vi "NavbalLabVIEW(15-5-21).vi"() -> ()   [LabVIEW 2010] (continued)
  out "Marker Phase":sgl[][](array[numeric])
  in  "Marker Listbox":i32(listbox)
  out "Ref Pt Plot":sgl[][](array[numeric])
  in  "# Runs":dbl=15.0
  out "Predicted Phase":dbl[](array[numeric])
  out "Predicted Mag":dbl[](array[numeric])
  out "Port Output Data":string[][](array[string])
  out "Stbd Output Data":string[][](array[string])
  out "Excel Output Array":string[][](array[string])
  in  "Menu Button 6":bool
  in  "Menu Button 4":bool
  in  "Menu Button 5":bool
  in  "Menu Button 3":bool
  in  "Menu Button 2":bool
  in  "Menu Button 1":bool
  out "time string":string="6:13:31 AM"
  out "date string":string="3/22/2014"
  # "PORT"
  # "STARBOARD"
  # "120 Hz"
  # "60 Hz"
  # "Aft Turb"
  # "Aft Turb"
  # "Fwd Turb"
  # "Fwd Turb"
  # "Aft Gen"
  # "Aft Gen"
  # "Fwd Gen"
  # "Fwd Gen"
  # "NOTE: Use IMI Calibrator and\nmake sure dip switch in 'Peak' position"
  # "Simulated Signals Settings"
  # "NOTE: Each row is a different channel, columns correspond to rotational frequencies"
  # "NOTE: Each row is a different channel, columns correspond to rotational frequencies"
  # "NOTE: Each row is a different channel, columns correspond to rotational frequencies"
  # "NOTE: Each row is a different channel, columns correspond to rotational frequencies"
  # "FWD\nTURBINE"
  # "AFT \nGENERATOR"
  # "FWD\nGENERATOR"
  # "AFT\nTURBINE"
  # "START POINT"
  # "Weight"
  # "Location"
  # "Weight"
  # "Location"
  # "Weight"
  # "Location"
  # "Weight"
  # "Location"
  # "Weight"
  # "Location"
  # "Mag"
  # "Phase"
  # "Mag"
  # "Phase"
  # "Mag"
  # "Phase"
  # "Mag"
  # "Phase"
  # "Mag"
  # "Phase"
  # "Include how many runs in listbox?"
  # "3. Click \"Calculate Solution\"\n4. Double click desired solution option"
  # "1. Click  \"Calculate Response Coefficients\""
  # "2. Select Start Point"
  # "AT"
  # "AT"
  # "FT"
  # "FT"
  # "AG"
  # "AG"
  # "FG"
  # "FG"
  # "NET"
  # "Press to\nCalc Sum"
  # "AT"
  # "AT"
  # "AT"
  # "+"
  # "FT"
  # "FT"
  # "FT"
  # "LA: 10\nOhio: 2\nRig: 2 or 1"
  # "AG"
  # "AG"
  # "AG"
  # "FG"
  # "FG"
  # "FG"
  # "Sensor Weighting"
  # "AT              FT             AG             FG"
  # "AT             FT              AG             FG"
  # "Weight 1"
  # "Loc 2"
  # "Loc 1"
  # "Weight 2"
  # "Aft Turb"
  # "Fwd Turb"
  # "Aft Gen"
  # "Fwd Gen"
  # "Current"
  # "Marker"
  # "Solution"
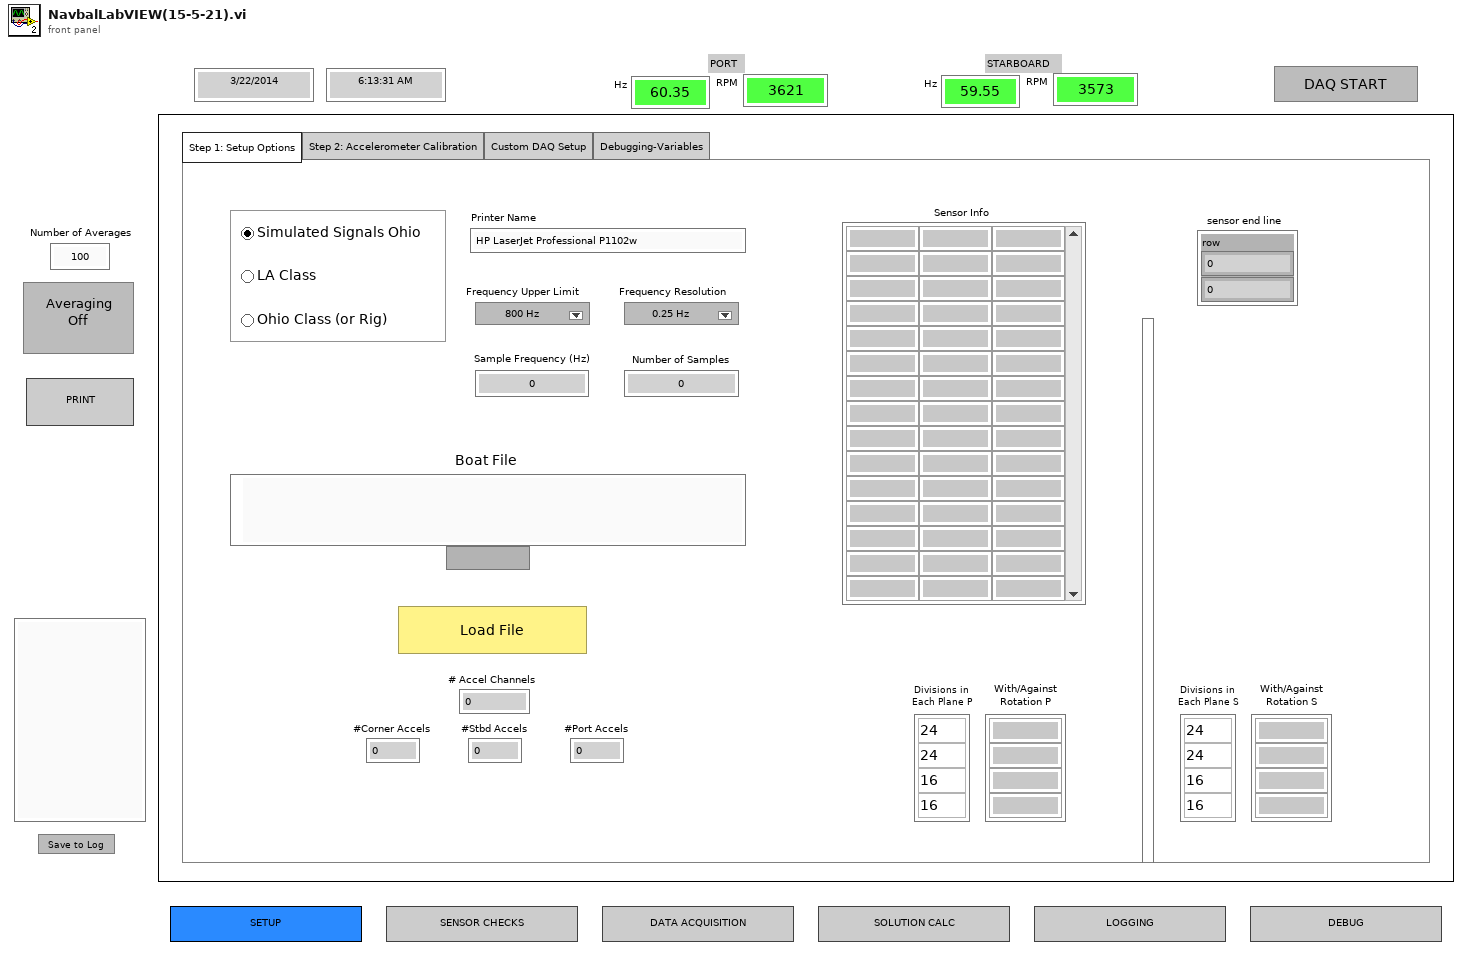
[diagram p1: front panel]
types:
  T1 = enum32{"Step 3: Background Checks", "Step 4: Sensor Overview", "Step 5: Vibration Survey", "Debugging - Indicators"}
  T2 = enum32{"Step 1: Setup Options", "Step 2: Accelerometer Calibration", "Custom DAQ Setup", "Debugging-Variables"}
  T3 = typedef "NI_Matrix.lvlib/RealMatrix.ctl" = dbl[][]
  T4 = enum32{"Simulated Signals Ohio", "LA Class", "Ohio Class"}
  T5 = cluster{"Amplitude":dbl, "Phase":dbl, "Amplitude 2":dbl, "Phase 2":dbl, "Amplitude 3":dbl, "Phase 3":dbl, "Amplitude 4":dbl, "Phase 4":dbl, "Amplitude 5":dbl, "Phase 5":dbl, "Amplitude 6":dbl, "Phase 6":dbl, "Amplitude 7":dbl, "Phase 7":dbl, "Amplitude 8":dbl, "Phase 8":dbl, "Amplitude 9":dbl, "Phase 9":dbl, "Amplitude 10":dbl, "Phase 10":dbl, "Amplitude 11":dbl, "Phase 11":dbl, "Amplitude 12":dbl, "Phase 12":dbl}
  T6 = cluster{"Frequency":dbl, "Amplitude":dbl, "Amplitude 2":dbl, "Amplitude 3":dbl, "Amplitude 4":dbl, "Amplitude 5":dbl, "Amplitude 6":dbl, "Amplitude 7":dbl, "Amplitude 8":dbl, "Amplitude 9":dbl, "Phase":dbl, "Phase 2":dbl, "Phase 3":dbl, "Phase 4":dbl, "Phase 5":dbl, "Phase 6":dbl, "Phase 7":dbl, "Phase 8":dbl, "Phase 9":dbl}
  T7 = enum32{"Other Adjustments", "Data Array STBD", "Data Array Port", "Data Array Corners-Stbd", "Data Array Corners-Port", "Solution Indicators", "Other Variables"}
  T8 = enum32{"Step 1: Response Coeff Variables", "Step 2: Calculate Goodman Solution", "Step 3: Optimal Balance Move", "Options", "Variables-For Reference"}
  T9 = enum32{"Step 6: Polar Plots", "Options", "Data Arrays"}
  T10 = cluster{"maximum":dbl, "minimum":dbl, "clip to min":bool, "log?(F)":bool, "grid color":u32, "plot color":u32, "fmt and prec":cluster{"format":enum8{"Decimal", "Scientific", "Engineering", "Binary", "Octal", "Hex"}, "precision":u8}, "visible section":u16}
  T11 = enum16{"Standard Report", "HTML", "Word", "Excel"}
  T12 = typedef "NI_ReportGenerationCore.lvlib/HTML Report Image Alignment.ctl" = enum16{"(default)", "LEFT", "RIGHT", "TOP", "TEXTTOP", "MIDDLE", "ABSMIDDLE", "BASELINE", "BOTTOM", "ABSBOTTOM"}
  T13 = cluster{"top":dbl, "left":dbl, "right":dbl, "bottom":dbl}
  T14 = cluster{"position (Excel)":cluster{"row":i32, "column":i32}, "name (Excel)":string, "bookmark (Word)":string}
  T15 = typedef "NI_Matrix.lvlib/ComplexMatrix.ctl" = cdb[][]
  T16 = enum8{"Enabled", "Disabled", "Disabled and Grayed Out"}
  T17 = typedef "Circular Buffer.lvlib/Circular Buffer Operations.ctl" = enum16{"Initialize", "Get Backlog", "Write", "Read (continuous)", "Read (most recent)"}
  T18 = typedef "NI_ReportGenerationToolkit.lvlib/font.ctl" = cluster{"font name":string, "font size":dbl, "bold":u16, "italic":u16, "underline":u16, "strike through":u16, "font color":u32}
  T19 = enum32{"Step 6: Polar Plots", "Data Arrays", "Options"}
  T20 = enum32{"Step 3: Sensor Overview", "Step 4: Background Checks", "Step 5: Vibration Survey", "Debugging - Indicators"}
  T21 = enum16{"User-specified Font", "Application Font", "System Font", "Dialog Font"}
  T22 = cluster{"Real Matrix Element":dbl, "Real Matrix Element":dbl}
  T23 = cluster{"Real Matrix Element":dbl, "Real Matrix Element":dbl}[]
  T24 = cluster{"Samples per Channel":u32, "# Accel Channels":i32}
diagram:
  w9 = u32 16252832
  # "random UI elements"
  # "Selection Color for Listbox"
  # "Default Booleans on Start"
  # "TODO:\nAdd Corner Pickups to both Starboard and Port Accel Arrays\n\nEdit Solution Permutation Structures for <4 plane Solutions\n\nAllow Solution Indicators to automatically grow to required dimensions as values are passed to them (Weights, Response Coeff, Prediction, etc.)\n\nMoving average indicator for last Scans, so that we can see more of the past scans\n->Add a Control for number of runs to average per point\n\nFull Implementation / Memory of recent Starboard and Port Baselines and Effects\n\nAllow Frequency indicator to update faster\n\n10/24/14\n- transferred from this computer to the Dell 1 computer (primary navbal computer)\n-"
  n1 = while {
    stop <- "stop 4" stop-if-true
    # "Event Structure: Button Nodes, Printer"
    n2 = control-ref of="Tab 1"() -> (w26:refnum<vi>)
    n3 = control-ref of="Tab 2"() -> (w13:refnum<vi>)
    n4 = control-ref of="Tab 3"() -> (w25:refnum<vi>)
    n5 = control-ref of="Tab 4"() -> (w24:refnum<vi>)
    n6 = control-ref of="Tab 5"() -> (w23:refnum<vi>)
    n7 = control-ref of="Tab 6"() -> (w22:refnum<vi>)
    n8 = Wait (ms)(milliseconds to wait=u32 500) -> ()  [unwired: 1 out]
    n9 = control-ref of="Menu Button 1"() -> (w21:refnum<vi>)
    n10 = control-ref of="Menu Button 2"() -> (w20:refnum<vi>)
    n11 = control-ref of="Menu Button 3"() -> (w19:refnum<vi>)
    n12 = control-ref of="Menu Button 5"() -> (w18:refnum<vi>)
    n13 = control-ref of="Menu Button 4"() -> (w17:refnum<vi>)
    n14 = control-ref of="Menu Button 6"() -> (w16:refnum<vi>)
    n15 = event shown="[4] \"Solution Options\": Value Change" {
      selector: _ -> [_ _ _ _ _ _ _ _ _ _ _ _ _ _ _ _ _ _]
      dyn-events: _ -> [_ _ _ _ _ _ _ _ _ _ _ _ _ _ _ _ _ _]
      timeout: _ -> [_ _ _ _ _ _ _ _ _ _ _ _ _ _ _ _ _ _]
      tunnel: w26 -> [w37 w57 w77 w97 _ _ _ _ _ _ _ w206 w225 w252 _ _ _ _]
      tunnel: w25 -> [w46 w66 w86 w106 _ _ _ _ _ _ _ w215 w235 w250 _ _ _ _]
      tunnel: w24 -> [w45 w65 w85 w105 _ _ _ _ _ _ _ w214 w234 w249 _ _ _ _]
      tunnel: w23 -> [w44 w64 w84 w104 _ _ _ _ _ _ _ w213 w233 w248 _ _ _ _]
      tunnel: w22 -> [w43 w63 w83 w103 _ _ _ _ _ _ _ w212 w232 w247 _ _ _ _]
      tunnel: w21 -> [w34 w56 w76 w96 _ _ _ _ _ _ _ w205 w224 _ _ _ _ _]
      tunnel: w20 -> [w33 w55 w75 w95 _ _ _ _ _ _ _ w204 w223 _ _ _ _ _]
      tunnel: w19 -> [w32 w54 w74 w94 _ _ _ _ _ _ _ w203 w222 _ _ _ _ _]
      tunnel: w18 -> [w31 w53 w73 w93 _ _ _ _ _ _ _ w202 w221 _ _ _ _ _]
      tunnel: w17 -> [w30 w52 w72 w92 _ _ _ _ _ _ _ w201 w220 _ _ _ _ _]
      tunnel: w16 -> [w29 w51 w71 w91 _ _ _ _ _ _ _ w200 w219 _ _ _ _ _]
      tunnel: "Printer Name" -> [_ _ _ _ _ _ _ _ _ _ _ _ _ w266 _ _ _ _]
      tunnel: w13 -> [w27 w47 w67 w87 _ _ _ _ _ _ _ w196 w216 w251 _ _ _ _]
      event "Menu Button 1": Value Change {
        w35 = cluster{u32, u32}[] [{6579300, 13421772}] ("Colors [4]")
        n16 = event-data() -> ()  [unwired: 1 in, 5 out]
        n17 = property on="Property Node" class="TabCtl (strict)"(reference=w43, "Visible"=FALSE) -> ()  [unwired: 1 in, 2 out]
        n18 = property on="Property Node" class="TabCtl (strict)"(reference=w44, "Visible"=FALSE) -> ()  [unwired: 1 in, 2 out]
        n19 = property on="Property Node" class="TabCtl (strict)"(reference=w37, "Visible"=TRUE) -> ()  [unwired: 1 in, 2 out]
        n20 = property on="Property Node" class="TabCtl (strict)"(reference=w45, "Visible"=FALSE) -> ()  [unwired: 1 in, 2 out]
        n21 = property on="Property Node" class="TabCtl (strict)"(reference=w27, "Visible"=FALSE) -> ()  [unwired: 1 in, 2 out]
        n22 = property on="Property Node" class="TabCtl (strict)"(reference=w46, "Visible"=FALSE) -> ()  [unwired: 1 in, 2 out]
        n23 = property on="Property Node" class="Bool"(reference=w34, "Colors [4]"=cluster{u32, u32}[] [{0, 2788095}, {0, 0}, {0, 11513775}, {0, 0}]) -> ()  [unwired: 1 in, 2 out]
        n24 = property on="Property Node" class="Bool"(reference=w31, "Colors [4]"=w35) -> ()  [unwired: 1 in, 2 out]
        n25 = property on="Property Node" class="Bool"(reference=w30, "Colors [4]"=w35) -> ()  [unwired: 1 in, 2 out]
        n26 = property on="Property Node" class="Bool"(reference=w29, "Colors [4]"=w35) -> ()  [unwired: 1 in, 2 out]
        n27 = property on="Property Node" class="Bool"(reference=w33, "Colors [4]"=w35) -> ()  [unwired: 1 in, 2 out]
        n28 = property on="Property Node" class="Bool"(reference=w32, "Colors [4]"=w35) -> ()  [unwired: 1 in, 2 out]
      }
      event "Menu Button 2": Value Change {
        w49 = cluster{u32, u32}[] [{6579300, 13421772}] ("Colors [4]")
        n29 = event-data() -> ()  [unwired: 1 in, 5 out]
        n30 = property on="Property Node" class="TabCtl (strict)"(reference=w63, "Visible"=FALSE) -> ()  [unwired: 1 in, 2 out]
        n31 = property on="Property Node" class="TabCtl (strict)"(reference=w64, "Visible"=FALSE) -> ()  [unwired: 1 in, 2 out]
        n32 = property on="Property Node" class="TabCtl (strict)"(reference=w57, "Visible"=FALSE) -> ()  [unwired: 1 in, 2 out]
        n33 = property on="Property Node" class="TabCtl (strict)"(reference=w47, "Visible"=TRUE) -> ()  [unwired: 1 in, 2 out]
        n34 = property on="Property Node" class="TabCtl (strict)"(reference=w65, "Visible"=FALSE) -> ()  [unwired: 1 in, 2 out]
        n35 = property on="Property Node" class="TabCtl (strict)"(reference=w66, "Visible"=FALSE) -> ()  [unwired: 1 in, 2 out]
        n36 = property on="Property Node" class="Bool"(reference=w56, "Colors [4]"=w49) -> ()  [unwired: 1 in, 2 out]
        n37 = property on="Property Node" class="Bool"(reference=w53, "Colors [4]"=w49) -> ()  [unwired: 1 in, 2 out]
        n38 = property on="Property Node" class="Bool"(reference=w52, "Colors [4]"=w49) -> ()  [unwired: 1 in, 2 out]
        n39 = property on="Property Node" class="Bool"(reference=w55, "Colors [4]"=cluster{u32, u32}[] [{0, 16753194}, {0, 0}, {0, 11513775}, {0, 0}]) -> ()  [unwired: 1 in, 2 out]
        n40 = property on="Property Node" class="Bool"(reference=w51, "Colors [4]"=w49) -> ()  [unwired: 1 in, 2 out]
        n41 = property on="Property Node" class="Bool"(reference=w54, "Colors [4]"=w49) -> ()  [unwired: 1 in, 2 out]
      }
      event "Menu Button 3": Value Change {
        w69 = cluster{u32, u32}[] [{6579300, 13421772}] ("Colors [4]")
        n42 = event-data() -> ()  [unwired: 1 in, 5 out]
        n43 = property on="Property Node" class="TabCtl (strict)"(reference=w83, "Visible"=FALSE) -> ()  [unwired: 1 in, 2 out]
        n44 = property on="Property Node" class="TabCtl (strict)"(reference=w84, "Visible"=FALSE) -> ()  [unwired: 1 in, 2 out]
        n45 = property on="Property Node" class="TabCtl (strict)"(reference=w77, "Visible"=FALSE) -> ()  [unwired: 1 in, 2 out]
        n46 = property on="Property Node" class="TabCtl (strict)"(reference=w85, "Visible"=FALSE) -> ()  [unwired: 1 in, 2 out]
        n47 = property on="Property Node" class="TabCtl (strict)"(reference=w67, "Visible"=FALSE) -> ()  [unwired: 1 in, 2 out]
        n48 = property on="Property Node" class="TabCtl (strict)"(reference=w86, "Visible"=TRUE) -> ()  [unwired: 1 in, 2 out]
        n49 = property on="Property Node" class="Bool"(reference=w76, "Colors [4]"=w69) -> ()  [unwired: 1 in, 2 out]
        n50 = property on="Property Node" class="Bool"(reference=w73, "Colors [4]"=w69) -> ()  [unwired: 1 in, 2 out]
        n51 = property on="Property Node" class="Bool"(reference=w72, "Colors [4]"=w69) -> ()  [unwired: 1 in, 2 out]
        n52 = property on="Property Node" class="Bool"(reference=w75, "Colors [4]"=w69) -> ()  [unwired: 1 in, 2 out]
        n53 = property on="Property Node" class="Bool"(reference=w71, "Colors [4]"=w69) -> ()  [unwired: 1 in, 2 out]
        n54 = property on="Property Node" class="Bool"(reference=w74, "Colors [4]"=cluster{u32, u32}[] [{0, 16025855}, {0, 0}, {0, 11513775}, {0, 0}]) -> ()  [unwired: 1 in, 2 out]
      }
      event "Menu Button 4": Value Change {
        w90 = cluster{u32, u32}[] [{6579300, 13421772}] ("Colors [4]")
        n55 = event-data() -> ()  [unwired: 1 in, 5 out]
        n56 = property on="Property Node" class="TabCtl (strict)"(reference=w103, "Visible"=FALSE) -> ()  [unwired: 1 in, 2 out]
        n57 = property on="Property Node" class="TabCtl (strict)"(reference=w104, "Visible"=TRUE) -> ()  [unwired: 1 in, 2 out]
        n58 = property on="Property Node" class="TabCtl (strict)"(reference=w97, "Visible"=FALSE) -> ()  [unwired: 1 in, 2 out]
        n59 = property on="Property Node" class="TabCtl (strict)"(reference=w87, "Visible"=FALSE) -> ()  [unwired: 1 in, 2 out]
        n60 = property on="Property Node" class="TabCtl (strict)"(reference=w105, "Visible"=FALSE) -> ()  [unwired: 1 in, 2 out]
        n61 = property on="Property Node" class="TabCtl (strict)"(reference=w106, "Visible"=FALSE) -> ()  [unwired: 1 in, 2 out]
        n62 = property on="Property Node" class="Bool"(reference=w96, "Colors [4]"=w90) -> ()  [unwired: 1 in, 2 out]
        n63 = property on="Property Node" class="Bool"(reference=w93, "Colors [4]"=w90) -> ()  [unwired: 1 in, 2 out]
        n64 = property on="Property Node" class="Bool"(reference=w92, "Colors [4]"=cluster{u32, u32}[] [{0, 2853120}, {0, 0}, {0, 11513775}, {0, 0}]) -> ()  [unwired: 1 in, 2 out]
        n65 = property on="Property Node" class="Bool"(reference=w95, "Colors [4]"=w90) -> ()  [unwired: 1 in, 2 out]
        n66 = property on="Property Node" class="Bool"(reference=w91, "Colors [4]"=w90) -> ()  [unwired: 1 in, 2 out]
        n67 = property on="Property Node" class="Bool"(reference=w94, "Colors [4]"=w90) -> ()  [unwired: 1 in, 2 out]
      }
      event "Solution Options": Value Change {
        w107 = string[][] []
        w108 = csg[] [] ("AT Exceptions")
        n68 = event-data() -> ()  [unwired: 1 in, 5 out]
        n69 = property on="Aft Turbine Balance Plane Split Options" class="MCListbox (strict)"("ItemNames"=w107) -> ()  [unwired: 2 in, 2 out]
        n70 = property on="Fwd Turbine Balance Plane Split Options" class="MCListbox (strict)"("ItemNames"=w107) -> ()  [unwired: 2 in, 2 out]
        n71 = for {
          N: 50 -> [_]
          i -> [w112]
          n72 = Bundle(w112, "Column"=3) -> (w111:cluster{i32, "Column":i32})  [unwired: 1 in]
          n73 = property on="Prediction Results" class="MCListbox (strict)"("ActiveCell"=w111) -> ()  [unwired: 2 in, 2 out]
          n74 = property on="Prediction Results" class="MCListbox (strict)"("CellBG"=u32 16777215) -> ()  [unwired: 2 in, 2 out]
        }
        n75 = property on="Solution Options" class="MCListbox (strict)"("SelColor"=u32 2771455) -> ()  [unwired: 2 in, 2 out]
        n76 = property on="Fwd Generator Balance Plane Split Options" class="MCListbox (strict)"("ItemNames"=w107) -> ()  [unwired: 2 in, 2 out]
        n77 = property on="Aft Generator Balance Plane Split Options" class="MCListbox (strict)"("ItemNames"=w107) -> ()  [unwired: 2 in, 2 out]
        n78 = local write "AT Exceptions"(w108) -> ()
        n79 = local write "FT Exceptions"(w108) -> ()
        n80 = local write "AG Exceptions"(w108) -> ()
        n81 = local write "FG Exceptions"(w108) -> ()
      }
      event "Weight Category AT": Value Change {
        n82 = event-data() -> ()  [unwired: 1 in, 5 out]
      }
      event "MagPhase": Mouse Down {
        n83 = event-data() -> ()  [unwired: 1 in, 7 out]
        n84 = for {
          N: 60 -> [_]
          i -> [w116]
          n85 = flat-sequence {
            tunnel: w116 -> [w119]
            frame #0 {
              n86 = Bundle(w119, 5) -> (w117:cluster{i32, i32})  [unwired: 1 in]
              n87 = property on="MagPhase" class="MCListbox (strict)"("ActiveCell"=w117) -> ()  [unwired: 2 in, 2 out]
            }
            frame #1 {
              n88 = property on="MagPhase" class="MCListbox (strict)"("CellBG"=u32 16777215) -> ()  [unwired: 2 in, 2 out]
            }
          }
        }
      }
      event "Weight Category FT": Value Change {
        n89 = event-data() -> ()  [unwired: 1 in, 5 out]
      }
      event "Weight Category AG": Value Change {
        n90 = event-data() -> ()  [unwired: 1 in, 5 out]
      }
      event "Weight Category FG": Value Change {
        n91 = event-data() -> ()  [unwired: 1 in, 5 out]
      }
      event "Load File": Value Change {
        w144 = 0
        # "Whether Planes are with or Against \nRotation"
        # "Number of Balance Plane Divisions:\n3rd tab 2nd row"
        # "Sensor info: Pick up the first \n3 columns from the  4th tab in Excel"
        n92 = event-data() -> ()  [unwired: 1 in, 5 out]
        n93 = property on="Boat File" class="Path"() -> ("Value"=w164:path)  [unwired: 2 in, 2 out]
        n94 = call <vilib>:"New Report.vi"("report type"=T11."Excel", "template (empty)"=w164) -> ("report out"=w157:refnum<class "NI_report.lvclass">, "error out"=w156:errorcluster)  [unwired: 12 in]
        n95 = call <vilib>:"Excel Get Worksheet.vi"("report in"=w157, "worksheet index (0)"=2, "error in (no error)"=w156) -> ("report out"=w136:refnum<class "NI_report.lvclass">, "error out"=w135:errorcluster)  [unwired: 11 out]
        n96 = call <vilib>:"Excel Get Worksheet.vi"("report in"=w157, "worksheet index (0)"=3, "error in (no error)"=w156) -> ("report out"=w152:refnum<class "NI_report.lvclass">, "error out"=w151:errorcluster)  [unwired: 11 out]
        n97 = call <vilib>:"Excel Get Last Row.vi"("report in"=w152, "error in (no error)"=w151) -> ("report out"=w160:refnum<class "NI_report.lvclass">, "MS Office parameters out"=w170:T14, "error out"=w159:errorcluster)  [unwired: 11 in]
        n98 = call-poly <vilib>:"Excel Get Data.vi"("report in"=w136, "data type"=string[][] [], "start (-1, -1)"=cluster{"row":i32, "column":i32} {"row"=2, "column"=1}, "end (-1, -1)"=cluster{"row":i32, "column":i32} {"row"=2, "column"=8} ("start (-1, -1)"), "error in (no error)"=w135) -> ("data"=w131:string[][])  [unwired: 10 out]
        n99 = call-poly <vilib>:"Excel Get Data.vi"("report in"=w136, "data type"=i32[][] [], "start (-1, -1)"=cluster{"row":i32, "column":i32} {"row"=1, "column"=1}, "end (-1, -1)"=cluster{"row":i32, "column":i32} {"row"=1, "column"=8} ("start (-1, -1)"), "error in (no error)"=w135) -> ("data"=w145:i32[][])  [unwired: 10 out]
        n100 = Unbundle(w170) -> ("position (Excel)"=w169:cluster{"row":i32, "column":i32})  [unwired: 2 out]
        n101 = Transpose 2D Array(2D array=w131) -> (transposed array=w126:string[][])
        n102 = Transpose Matrix(1:w145) -> (0:w130:dbl[][])
        n103 = Unbundle(w169) -> ("row"=w168:i32)  [unwired: 1 out]
        n104 = Decrement(x=w168) -> (x-1=w150:i32)
        n105 = Delete From Array(array=w130, length=4, index (row)=4 ("disabled index (col)")) -> (deleted portion=w128:dbl[][], array with subset deleted=w121:dbl[][])  [unwired: 1 in]
        n106 = Delete From Array(array=w126, length=4, index (row)=4 ("disabled index (col)")) -> (deleted portion=→"With/Against\nRotation S":string[][], array with subset deleted=→"With/Against\nRotation P":string[][])  [unwired: 1 in]
        n107 = Bundle(w150, 2) -> (w162:cluster{i32, i32})  [unwired: 1 in]
        "sensor end line" <- w162
        n108 = call-poly <vilib>:"Excel Get Data.vi"("report in"=w160, "data type"=string[][] [], "start (-1, -1)"=cluster{"row":i32, "column":i32} {"row"=1, "column"=0}, "end (-1, -1)"=w162, "error in (no error)"=w159) -> ("data"=w143:string[][], "error out"=w161:errorcluster)  [unwired: 9 out]
        "Sensor Info" <- w143
        n109 = call <vilib>:"General Error Handler.vi"("error in (no error)"=w161) -> ()  [unwired: 2 in, 13 out]
        n110 = Array Size(array=w143) -> (size(s)=w148:i32[])
        n111 = Array Size(array=w143) -> (size(s)=w142:i32[])
        n112 = Index Array(array=w148, index=0) -> (element=→"# Accel Channels":i32)
        n113 = property on="Divisions in\nEach Plane S" class="Arr (strict)"("Value"=w128) -> ()  [unwired: 2 in, 2 out]
        n114 = property on="Divisions in\nEach Plane P" class="Arr (strict)"("Value"=w121) -> ()  [unwired: 2 in, 2 out]
        n115 = Index Array(array=w142, index=0) -> (element=w140:i32)
        n116 = for {
          N: w140 -> [_]
          tunnel: w143 -> [w186]
          shift-right: [w180] -> w139
          shift-left: w144 -> [w181]
          shift-right: [w176] -> w138
          shift-left: w144 -> [w177]
          shift-right: [w174] -> w137
          shift-left: w144 -> [w175]
          i -> [w184]
          n117 = Index Array(array=w186, index (row)=w184, index (col)=2 ("disabled index (col)")) -> (element=w171:string)
          n118 = Equal?(x=w171, y="Corner") -> (x = y?=w182:bool)
          n119 = Equal?(x=w171, y="Stbd Brng") -> (x = y?=w178:bool)
          n120 = Equal?(x=w171, y="Port Brng") -> (x = y?=w172:bool)
          n121 = case shown="True" w182 {
            tunnel: w181 -> [w193 w195]
            tunnel: [w193 w194] -> w180
            frame False {
            }
            frame True {
              n122 = Increment(x=w195) -> (x+1=w194:i32)
            }
          }
          n123 = case shown="True" w178 {
            tunnel: [w190 w192] -> w176
            tunnel: w177 -> [w190 w191]
            frame False {
            }
            frame True {
              n124 = Increment(x=w191) -> (x+1=w192:i32)
            }
          }
          n125 = case shown="True" w172 {
            tunnel: [w187 w189] -> w174
            tunnel: w175 -> [w187 w188]
            frame False {
            }
            frame True {
              n126 = Increment(x=w188) -> (x+1=w189:i32)
            }
          }
        }
        "#Corner Accels" <- w139
        "#Stbd Accels" <- w138
        "#Port Accels" <- w137
      }
      event "Menu Button 5": Value Change {
        w199 = cluster{u32, u32}[] [{6579300, 13421772}] ("Colors [4]")
        n127 = event-data() -> ()  [unwired: 1 in, 5 out]
        n128 = property on="Property Node" class="TabCtl (strict)"(reference=w212, "Visible"=FALSE) -> ()  [unwired: 1 in, 2 out]
        n129 = property on="Property Node" class="TabCtl (strict)"(reference=w213, "Visible"=FALSE) -> ()  [unwired: 1 in, 2 out]
        n130 = property on="Property Node" class="TabCtl (strict)"(reference=w206, "Visible"=FALSE) -> ()  [unwired: 1 in, 2 out]
        n131 = property on="Property Node" class="TabCtl (strict)"(reference=w214, "Visible"=TRUE) -> ()  [unwired: 1 in, 2 out]
        n132 = property on="Property Node" class="TabCtl (strict)"(reference=w196, "Visible"=FALSE) -> ()  [unwired: 1 in, 2 out]
        n133 = property on="Property Node" class="TabCtl (strict)"(reference=w215, "Visible"=FALSE) -> ()  [unwired: 1 in, 2 out]
        n134 = property on="Property Node" class="Bool"(reference=w205, "Colors [4]"=w199) -> ()  [unwired: 1 in, 2 out]
        n135 = property on="Property Node" class="Bool"(reference=w202, "Colors [4]"=cluster{u32, u32}[] [{0, 13696881}, {0, 0}, {0, 11513775}, {0, 0}]) -> ()  [unwired: 1 in, 2 out]
        n136 = property on="Property Node" class="Bool"(reference=w201, "Colors [4]"=w199) -> ()  [unwired: 1 in, 2 out]
        n137 = property on="Property Node" class="Bool"(reference=w204, "Colors [4]"=w199) -> ()  [unwired: 1 in, 2 out]
        n138 = property on="Property Node" class="Bool"(reference=w200, "Colors [4]"=w199) -> ()  [unwired: 1 in, 2 out]
        n139 = property on="Property Node" class="Bool"(reference=w203, "Colors [4]"=w199) -> ()  [unwired: 1 in, 2 out]
      }
      event "Menu Button 6": Value Change {
        w218 = cluster{u32, u32}[] [{6579300, 13421772}] ("Colors [4]")
        n140 = event-data() -> ()  [unwired: 1 in, 5 out]
        n141 = property on="Property Node" class="TabCtl (strict)"(reference=w232, "Visible"=TRUE) -> ()  [unwired: 1 in, 2 out]
        n142 = property on="Property Node" class="TabCtl (strict)"(reference=w233, "Visible"=FALSE) -> ()  [unwired: 1 in, 2 out]
        n143 = property on="Property Node" class="TabCtl (strict)"(reference=w225, "Visible"=FALSE) -> ()  [unwired: 1 in, 2 out]
        n144 = property on="Property Node" class="TabCtl (strict)"(reference=w216, "Visible"=FALSE) -> ()  [unwired: 1 in, 2 out]
        n145 = property on="Property Node" class="TabCtl (strict)"(reference=w234, "Visible"=FALSE) -> ()  [unwired: 1 in, 2 out]
        n146 = property on="Property Node" class="TabCtl (strict)"(reference=w235, "Visible"=FALSE) -> ()  [unwired: 1 in, 2 out]
        n147 = property on="Property Node" class="Bool"(reference=w224, "Colors [4]"=w218) -> ()  [unwired: 1 in, 2 out]
        n148 = property on="Property Node" class="Bool"(reference=w221, "Colors [4]"=w218) -> ()  [unwired: 1 in, 2 out]
        n149 = property on="Property Node" class="Bool"(reference=w220, "Colors [4]"=w218) -> ()  [unwired: 1 in, 2 out]
        n150 = property on="Property Node" class="Bool"(reference=w223, "Colors [4]"=w218) -> ()  [unwired: 1 in, 2 out]
        n151 = property on="Property Node" class="Bool"(reference=w219, "Colors [4]"=cluster{u32, u32}[] [{0, 5888767}, {0, 0}, {0, 11513775}, {0, 0}]) -> ()  [unwired: 1 in, 2 out]
        n152 = property on="Property Node" class="Bool"(reference=w222, "Colors [4]"=w218) -> ()  [unwired: 1 in, 2 out]
      }
      event "Print Button": Value Change {
        w267 = 1 items=["portrait", "landscape"] ("orientation (portrait)")
        n153 = event-data() -> ()  [unwired: 1 in, 5 out]
        n154 = property on="Tab 1" class="TabCtl (strict)"() -> ("Visible"=w246:bool)  [unwired: 2 in, 2 out]
        n155 = property on="Tab 2" class="TabCtl (strict)"() -> ("Visible"=w245:bool)  [unwired: 2 in, 2 out]
        n156 = property on="Tab 3" class="TabCtl (strict)"() -> ("Visible"=w241:bool)  [unwired: 2 in, 2 out]
        n157 = property on="Tab 4" class="TabCtl (strict)"() -> ("Visible"=w242:bool)  [unwired: 2 in, 2 out]
        n158 = property on="Tab 5" class="TabCtl (strict)"() -> ("Visible"=w243:bool)  [unwired: 2 in, 2 out]
        n159 = property on="Tab 6" class="TabCtl (strict)"() -> ("Visible"=w244:bool)  [unwired: 2 in, 2 out]
        n160 = Build Array(w252, w251, w250, w249, w248, w247) -> (w238:refnum<vi>[])
        n161 = Build Array(w246, w245, w241, w242, w243, w244) -> (w240:bool[])
        n162 = call <vilib>:"New Report.vi"("report type"=T11."Standard Report") -> ("report out"=w274:refnum<class "NI_report.lvclass">, "error out"=w273:errorcluster)  [unwired: 13 in]
        n163 = Get Date/Time String(want seconds? (F)=TRUE) -> (date string=w256:string, time string=w255:string)  [unwired: 2 in]
        n164 = for {
          tunnel: w240 -> [w277] mode=indexing
          tunnel: [w275] -> w239 mode=indexing
          i -> [w276]
          n165 = case shown="True" w277 {
            tunnel: w276 -> [_ w279]
            tunnel: [-1 w279] -> w275
            frame False {
            }
            frame True {
            }
          }
        }
        n166 = Concatenate Strings(w256, " - " ("string"), w255) -> (w253:string)
        n167 = Array Max & Min(array=w239) -> (max value=w237:i32)  [unwired: 3 out]
        n168 = Index Array(array=w238, index=w237) -> (element=w236:refnum<vi>)
        n169 = call-dynamic "Append Control Image to Report.vi"("report in"=w274, "alignment (default)"=HTML_Report_Image_Alignment."MIDDLE", "ctrl reference"=w236, "error in (no error)"=w273) -> ("report out"=w269:refnum<class "NI_report.lvclass">, "error out"=w268:errorcluster)  [unwired: 8 in, 2 out]
        n170 = call-dynamic "Set Report Orientation.vi"("report in"=w269, "orientation (portrait)"=w267, "error in (no error)"=w268) -> ("report out"=w264:refnum<class "NI_report.lvclass">, "error out"=w265:errorcluster)  [unwired: 11 in]
        n171 = call-dynamic "Set Report Margins.vi"("report in"=w264, "margins (1.00)"=T13 {"top"=0.3, "left"=0.5, "right"=0.5, "bottom"=0.3}, "error in (no error)"=w265) -> ("report out"=w262:refnum<class "NI_report.lvclass">, "error out"=w261:errorcluster)  [unwired: 10 in, 1 out]
        n172 = call-dynamic "Set Report Footer Text.vi"("report in"=w262, "center footer text"=w253, "error in (no error)"=w261) -> ("report out"=w260:refnum<class "NI_report.lvclass">, "error out"=w259:errorcluster)  [unwired: 11 in]
        n173 = call-dynamic "Print Report.vi"("report in"=w260, "printer name (default)"=w266, "error in (no error)"=w259) -> ("report out"=w272:refnum<class "NI_report.lvclass">, "error out"=w271:errorcluster)  [unwired: 11 in]
        n174 = call-dynamic "Dispose Report.vi"("report in"=w272, "error in (no error)"=w271) -> ()  [unwired: 13 in, 1 out]
      }
      event "Aft Turbine Balance Plane Split Options": Value Change {
        n175 = event-data() -> ()  [unwired: 1 in, 5 out]
        n176 = for {
          N: 50 -> [_]
          i -> [w283]
          n177 = Bundle(w283, "Column"=3) -> (w282:cluster{i32, "Column":i32})  [unwired: 1 in]
          n178 = property on="Prediction Results" class="MCListbox (strict)"("ActiveCell"=w282) -> ()  [unwired: 2 in, 2 out]
          n179 = property on="Prediction Results" class="MCListbox (strict)"("CellBG"=u32 16777215) -> ()  [unwired: 2 in, 2 out]
        }
        n180 = property on="Aft Turbine Balance Plane Split Options" class="MCListbox (strict)"("SelColor"=u32 2771455) -> ()  [unwired: 2 in, 2 out]
      }
      event "Fwd Turbine Balance Plane Split Options": Value Change {
        n181 = event-data() -> ()  [unwired: 1 in, 5 out]
        n182 = for {
          N: 50 -> [_]
          i -> [w289]
          n183 = Bundle(w289, "Column"=3) -> (w288:cluster{i32, "Column":i32})  [unwired: 1 in]
          n184 = property on="Prediction Results" class="MCListbox (strict)"("ActiveCell"=w288) -> ()  [unwired: 2 in, 2 out]
          n185 = property on="Prediction Results" class="MCListbox (strict)"("CellBG"=u32 16777215) -> ()  [unwired: 2 in, 2 out]
        }
        n186 = property on="Fwd Turbine Balance Plane Split Options" class="MCListbox (strict)"("SelColor"=u32 2771455) -> ()  [unwired: 2 in, 2 out]
      }
      event "Aft Generator Balance Plane Split Options": Value Change {
        n187 = event-data() -> ()  [unwired: 1 in, 5 out]
        n188 = for {
          N: 50 -> [_]
          i -> [w295]
          n189 = Bundle(w295, "Column"=3) -> (w294:cluster{i32, "Column":i32})  [unwired: 1 in]
          n190 = property on="Prediction Results" class="MCListbox (strict)"("ActiveCell"=w294) -> ()  [unwired: 2 in, 2 out]
          n191 = property on="Prediction Results" class="MCListbox (strict)"("CellBG"=u32 16777215) -> ()  [unwired: 2 in, 2 out]
        }
        n192 = property on="Aft Generator Balance Plane Split Options" class="MCListbox (strict)"("SelColor"=u32 2771455) -> ()  [unwired: 2 in, 2 out]
      }
      event "Fwd Generator Balance Plane Split Options": Value Change {
        n193 = event-data() -> ()  [unwired: 1 in, 5 out]
        n194 = for {
          N: 50 -> [_]
          i -> [w301]
          n195 = Bundle(w301, "Column"=3) -> (w300:cluster{i32, "Column":i32})  [unwired: 1 in]
          n196 = property on="Prediction Results" class="MCListbox (strict)"("ActiveCell"=w300) -> ()  [unwired: 2 in, 2 out]
          n197 = property on="Prediction Results" class="MCListbox (strict)"("CellBG"=u32 16777215) -> ()  [unwired: 2 in, 2 out]
        }
        n198 = property on="Fwd Generator Balance Plane Split Options" class="MCListbox (strict)"("SelColor"=u32 2771455) -> ()  [unwired: 2 in, 2 out]
      }
    }
  }
  n199 = while {
    stop <- "stop 2" stop-if-true
    w305 = path "C:/Users/Jim Gehringer/Desktop/Navbal-LabVIEW_FINAL/Balancelog.txt" ("file (use dialog)")
    # "Logging"
    # "Time and Date"
    n200 = call <vilib>:"Check if File or Folder Exists.vi"("path"=w305) -> ("file or folder exists?"=w315:bool)  [unwired: 8 in, 2 out]
    n201 = Get Date/Time String(want seconds? (F)=TRUE) -> (date string=w304:string, time string=w316:string)  [unwired: 2 in]
    "date string" <- w304
    "time string" <- w316
    n202 = case shown="True" w315 {
      tunnel: w305 -> [_ w340]
      frame False {
      }
      frame True {
        n203 = Read from Text File(file (use dialog)=w340) -> (text=→"text":string)  [unwired: 3 in, 3 out]
      }
    }
    n204 = case shown="True" "Enter into log" {
      tunnel: w316 -> [_ w324]
      tunnel: w305 -> [_ w321]
      tunnel: w304 -> [_ w319]
      frame False {
      }
      frame True {
        n205 = call <vilib>:"Check if File or Folder Exists.vi"("path"=w321) -> ("file or folder exists?"=w323:bool)  [unwired: 8 in, 2 out]
        n206 = property on="Log Input" class="Str"("Value"="" ("Log Input")) -> ()  [unwired: 2 in, 2 out]
        n207 = case shown="True" w323 {
          tunnel: w321 -> [w327 w337]
          tunnel: w324 -> [w331 w334]
          tunnel: "Log Input" -> [w329 w336]
          tunnel: w319 -> [w325 w332]
          frame False {
            n208 = call <vilib>:"Space Constant.vi"() -> ("String"=w326:string)
            n209 = Concatenate Strings(w325, w326, w331, "\r", w329) -> (w328:string)
            n210 = Write to Text File(file (use dialog)=w327, text=w328) -> ()  [unwired: 2 in, 3 out]
          }
          frame True {
            w335 = "\r"
            n211 = call <vilib>:"Space Constant.vi"() -> ("String"=w333:string)
            n212 = Read from Text File(file (use dialog)=w337) -> (text=w339:string)  [unwired: 3 in, 3 out]
            n213 = Concatenate Strings(w339, w335, w335, w332, w333, w334, w335, w336) -> (w338:string)
            n214 = Write to Text File(file (use dialog)=w337, text=w338) -> ()  [unwired: 2 in, 3 out]
          }
        }
      }
    }
    n215 = Search and Replace String(replace all?=TRUE ("replace all? (F)"), input string=w304, search string="/" ("substring (\"\")"), replace string="-" ("replace string (\"\")")) -> (result string=w310:string)  [unwired: 4 in, 3 out]
    n216 = Path To String(path=w305) -> (string=w312:string)
    n217 = Concatenate Strings(w312, "\\" ("string"), w310, ".txt" ("string")) -> (w309:string)
    "Log File Path" <- w309
    n218 = String To Path(string=w309) -> ()  [unwired: 1 out]
  }
  n219 = property on="Calibration Channel List" class="MCListbox (strict)"() -> ("NumRows"=w6:u32)  [unwired: 2 in, 2 out]
  n220 = property on="Calibration Channel List" class="MCListbox (strict)"() -> ("ItemNames"=w5:string[][])  [unwired: 2 in, 2 out]
  n221 = for {
    N: w6 -> [_]
    i -> [w343]
    n222 = Bundle(w343, 2) -> (w342:cluster{i32, i32})  [unwired: 1 in]
    n223 = property on="Calibration Channel List" class="MCListbox (strict)"("ActiveCell"=w342) -> ()  [unwired: 2 in, 2 out]
    n224 = property on="Calibration Channel List" class="MCListbox (strict)"("CellBG"=u32 16777215) -> ()  [unwired: 2 in, 2 out]
  }
  n225 = local write "Marker Time"(" " ("Marker Time")) -> ()
  n226 = property on="DAQ Listbox" class="MCListbox (strict)"("SelColor"=w9) -> ()  [unwired: 2 in, 2 out]
  n227 = property on="MagPhase" class="MCListbox (strict)"("SelColor"=w9) -> ()  [unwired: 2 in, 2 out]
  n228 = property on="DAQ Start" class="Bool (strict)"("BoolText.Text"="DAQ START" ("Boolean Text.Text")) -> ()  [unwired: 2 in, 2 out]
  n229 = Replace Array Subset(array=w5, new element=string[] ["", "", "", "", "", "", "", "", "", "", "", "", "", "", "", "", "", "", "", "", "", "", "", "", "", "", "", "", "", "", "", "", "", "", "", "", "", "", "", "", " "] ("new element/subarray"), index (col)=2 ("disabled index (col)")) -> (w2:string[][])  [unwired: 1 in]
  n230 = property on="stop 2" class="Bool"("Visible"=FALSE) -> ()  [unwired: 2 in, 2 out]
  n231 = property on="stop 4" class="Bool"("Visible"=FALSE) -> ()  [unwired: 2 in, 2 out]
  n232 = property on="Calibration Channel List" class="MCListbox (strict)"("ItemNames"=w2) -> ()  [unwired: 2 in, 2 out]
  n233 = local write "DAQ Start"(FALSE ("Visible")) -> ()
  n234 = while {
    stop <- w374 stop-if-true
    # "Technically, the 7th tab is the Port \ndata tab, but the vis skip tabs that \nare charts"
    # "+2 to include tachs"
    # "Number of Samples"
    # "Sampling Rate"
    n235 = local read "# Accel Channels"() -> (w362:i32)
    n236 = local read "Number of Samples"() -> (w367:i32)
    n237 = Wait (ms)(milliseconds to wait=u32 200) -> ()  [unwired: 1 out]
    n238 = Add(x=w362, y=2) -> (x+y=w360:i32)
    n239 = case shown="2" "Frequency Upper Limit" {
      tunnel: [512 1024 2048 4096 8192 16384 32768] -> w369
      frame 0, Default {
      }
      frame 1 {
      }
      frame 2 {
      }
      frame 3 {
      }
      frame 4 {
      }
      frame 5 {
      }
      frame 6 {
      }
    }
    "Sample Frequency (Hz)" <- w369
    n240 = case shown="0, Default" "Frequency Resolution" {
      tunnel: w369 -> [w3249 w3252 w3255 w3258 w3261]
      tunnel: [w3247 w3250 w3253 w3256 w3259] -> w368
      frame 0, Default {
        n241 = Divide(x=w3249, y=sgl 0.25) -> (x/y=w3247:sgl)
      }
      frame 1 {
        n242 = Divide(x=w3252, y=sgl 0.5) -> (x/y=w3250:sgl)
      }
      frame 2 {
        n243 = Divide(x=w3255, y=sgl 1.0) -> (x/y=w3253:sgl)
      }
      frame 3 {
        n244 = Divide(x=w3258, y=sgl 5.0) -> (x/y=w3256:sgl)
      }
      frame 4 {
        n245 = Divide(x=w3261, y=sgl 10.0) -> (x/y=w3259:sgl)
      }
    }
    "Number of Samples" <- w368
    n246 = Bundle("Number of Samples"=w367, w360) -> (w366:cluster{"Number of Samples":i32, i32})  [unwired: 1 in]
    n247 = case "Start Data Acquisition" shown="True" "DAQ Start" {
      tunnel: [FALSE FALSE] -> w374
      tunnel: "Ship Class" -> [_ w3287]
      tunnel: w366 -> [w3271 w3282]
      frame False {
        n248 = call-poly <userlib>:"Circular Buffer.vi"("Buffer Size"=w3271, "error in (no error)"=errorcluster {"status"=FALSE, "code"=0, "source"=""}, "Operation"=Circular_Buffer_Operations."Initialize", "Data In"=waveform(dbl)[] []) -> ()  [unwired: 4 in, 4 out]
        n249 = local write "Marker Phase"(sgl[][] [] ("Marker Phase")) -> ()
        n250 = local write "Marker Mag"(sgl[][] [] ("Marker Mag")) -> ()
        n251 = property on="Accel Calib Start" class="Bool (strict)"("DisabledEnum"=T16."Enabled" ("Disabled")) -> ()  [unwired: 2 in, 2 out]
        n252 = property on="DAQ Start" class="Bool (strict)"("BoolText.Text"="DAQ START" ("Boolean Text.Text")) -> ()  [unwired: 2 in, 2 out]
      }
      frame True {
        w3279 = dbl[][][] []
        n253 = local read "Sample Frequency (Hz)"() -> (w3278:i32)
        n254 = local read "Sensor Info"() -> (w3286:string[][])
        n255 = property on="Accel Calib Start" class="Bool (strict)"("DisabledEnum"=T16."Disabled and Grayed Out" ("Disabled")) -> ()  [unwired: 2 in, 2 out]
        n256 = Index Array(array=w3286, index (col)=1 ("disabled index (col)")) -> (element=w3284:string[])  [unwired: 1 in]
        n257 = Fract/Exp String To Number(string=w3284, default (0 dbl)=sgl 0.0 ("default (0 DBL)")) -> (number=w3281:sgl[])  [unwired: 2 in, 1 out]
        n258 = case shown="\"Simulated Signals Ohio\"" w3287 {
          tunnel: w3282 -> [w3292 w3303 w3315]
          tunnel: w3282 -> [w3291 w3302 w3316]
          tunnel: w3281 -> [w3290 w3304 _]
          tunnel: w3278 -> [w3289 w3305 _]
          frame "Ohio Class" {
            n259 = call-poly <userlib>:"Circular Buffer.vi"("Buffer Size"=w3292, "Operation"=Circular_Buffer_Operations."Initialize") -> ()  [unwired: 6 in, 4 out]
            n260 = while {
              tunnel: w3291 -> [w3299]
              tunnel: w3289 -> [w3296]
              tunnel: w3290 -> [w3295]
              stop <- w3294 stop-if-true
              n261 = local read "DAQ Start"() -> (w3300:bool)
              n262 = Not(x=w3300) -> (.not. x?=w3294:bool)
              n263 = call "DAQAssist-Ohioclass.vi"("Calibration Array"=w3295, "number of samples"=64, "rate"=w3296, "stopped"=w3294) -> ("Dynamic Data Type"=w3298:dynamicdata)  [unwired: 1 in, 1 out]
              n264 = call-poly <userlib>:"Circular Buffer.vi"("Buffer Size"=w3299, "Operation"=Circular_Buffer_Operations."Write", "Data In"=w3298) -> ()  [unwired: 5 in, 4 out]
            }
          }
          frame "LA Class" {
            # "Initialize buffer, then start reading data into buffer"
            n265 = call-poly <userlib>:"Circular Buffer.vi"("Buffer Size"=w3303, "Operation"=Circular_Buffer_Operations."Initialize") -> ()  [unwired: 6 in, 4 out]
            n266 = while {
              tunnel: w3305 -> [w3309]
              tunnel: w3304 -> [w3311]
              tunnel: w3302 -> [w3310]
              stop <- w3307 stop-if-true
              n267 = local read "DAQ Start"() -> (w3313:bool)
              n268 = Not(x=w3313) -> (.not. x?=w3307:bool)
              n269 = call "DAQAssist-LAclass.vi"("Calibration Array"=w3311, "number of samples"=64, "rate"=w3309, "stopped"=w3307) -> ("Dynamic Data Type"=w3312:dynamicdata)  [unwired: 1 in, 1 out]
              n270 = call-poly <userlib>:"Circular Buffer.vi"("Buffer Size"=w3310, "Operation"=Circular_Buffer_Operations."Write", "Data In"=w3312) -> ()  [unwired: 5 in, 4 out]
            }
          }
          frame "Simulated Signals Ohio" {
            n271 = call-poly <userlib>:"Circular Buffer.vi"("Buffer Size"=w3315, "Operation"=Circular_Buffer_Operations."Initialize") -> ()  [unwired: 6 in, 4 out]
            n272 = while "Write data into buffer variable" {
              tunnel: w3316 -> [w3324]
              stop <- w3326 stop-if-true
              n273 = control-ref of="Sample Frequency (Hz)"() -> (w3323:refnum<vi>)
              n274 = call "DAQAssist-SimulatedSignal(Ohio).vi"("reference"=w3323, "Stbd Cluster"="Stbd Cluster", "Port Cluster"="Port Cluster", "Corner Cluster Stbd"="Corner Cluster Stbd", "Corner Cluster Port"="Corner Cluster Port") -> ("Dynamic Data"=w3320:dynamicdata)
              n275 = call-poly <userlib>:"Circular Buffer.vi"("Buffer Size"=w3324, "Operation"=Circular_Buffer_Operations."Write", "Data In"=w3320) -> ()  [unwired: 5 in, 4 out]
              n276 = local read "DAQ Start"() -> (w3325:bool)
              n277 = Not(x=w3325) -> (.not. x?=w3326:bool)
            }
          }
        }
        n278 = while "Start reading buffer values and computing Magnitude and Phase" {
          shift-right: [w3474] -> _
          shift-left: w3279 -> [w3333]
          shift-right: [w3344] -> _
          shift-left: w3279 -> [w3332]
          shift-right: [w3473] -> _
          shift-left: w3279 -> [w3331]
          tunnel: w3287 -> [w3369]
          tunnel: w3282 -> [w3530]
          shift-right: [w3472] -> _
          shift-left: w3279 -> [w3330]
          stop <- w3567 stop-if-true
          # "Stbd Bearings"
          # "Port Bearings"
          # "Stbd Corners"
          # "Port Corners"
          # "Stbd Bearings"
          # "Port Bearings"
          # "Stbd Corners"
          # "Port Corners"
          # "Order of graphs\nin vibration survey selector"
          # "Using the Extract Tone VI, find the largest tone \nexhibited in the tach signal"
          # "Read and save 600 points"
          # "DATA ACQUISITION TAB"
          # "DATA ACQUISITION TAB"
          # "DATA ACQUISITION TAB"
          # "DATA ACQUISITION TAB"
          # "DATA ACQUISITION TAB"
          # "Vibration Survey Tab"
          # "Omit Tach"
          # "Omit Tach"
          # "Corners"
          # "Port"
          # "Stbd"
          # "Pick out first rotation"
          # "Array: Channel,Mils/sec,Phase,AdB,Mils(1x)"
          # "Measure Mils"
          # "Measure Magnitude"
          # "Measure Phase"
          # "Scan Data"
          # "Pick out first rotation"
          # "Array: Channel,Mils/sec,Phase,AdB,Mils(1x)"
          # "Measure Mils"
          # "Measure Magnitude"
          # "Measure Phase"
          # "Pick out first rotation"
          # "Array: Channel,Mils/sec,Phase,AdB,Mils(1x)"
          # "Measure Mils"
          # "Measure Magnitude"
          # "Measure Phase"
          # "Frequency Output"
          # "Array: Channel,Mils/sec,Phase,AdB,Mils(1x)"
          # "Measure Mils"
          # "Accels only"
          # "Measure Magnitude"
          # "Measure Phase"
          n279 = property on="Tab 2" class="TabCtl (strict)"() -> ("Value"=w3455:T1)  [unwired: 2 in, 2 out]
          n280 = property on="Tab 2" class="TabCtl (strict)"() -> ("Visible"=w3448:bool)  [unwired: 2 in, 2 out]
          n281 = Equal?(x=w3455, y=T1."Step 3: Background Checks") -> (x = y?=w3449:bool)
          n282 = local read "DAQ Start"() -> (w3568:bool)
          n283 = And(x=w3449, y=w3448) -> (x .and. y?=w3447:bool)
          n284 = case shown="True" w3447 {
            tunnel: w3369 -> [_ w4086]
            frame False {
            }
            frame True {
              # "Background Check"
              n285 = local read "Sensor Info"() -> (w4088:string[][])
              n286 = local read "AdB Starboard"() -> (w4115:cluster{"x0":dbl, "dx":dbl, dbl[][]})
              n287 = local read "AdB Port"() -> (w4116:cluster{"x0":dbl, "dx":dbl, dbl[][]})
              n288 = local read "AdB Corners"() -> (w4114:cluster{"x0":dbl, "dx":dbl, dbl[][]})
              n289 = local read "frequency resolution"() -> (w4109:dbl)
              n290 = property on="XY Graph" class="XYGraph (strict)"() -> ("Cursor.Cursor X"=w4097:dbl)  [unwired: 2 in, 2 out]
              n291 = Unbundle(w4115) -> (w4106:dbl[][])  [unwired: 2 out]
              n292 = Unbundle(w4114) -> (w4105:dbl[][])  [unwired: 2 out]
              n293 = Unbundle(w4116) -> (w4107:dbl[][])  [unwired: 2 out]
              n294 = Index Array(array=w4088, index (col)=0 ("disabled index (col)")) -> (element=w4087:string[])  [unwired: 1 in]
              n295 = local read "frequency resolution"() -> (w4113:dbl)
              n296 = Decrement(x=w4097) -> (x-1=w4096:dbl)
              n297 = Index Array(array=w4087, index=w4096) -> (element=→"Sensor Name":string)
              n298 = Divide(x=120.0, y=w4109) -> (x/y=w4108:dbl)
              n299 = Divide(x=60.0, y=w4113) -> (x/y=w4111:dbl)
              n300 = Index Array(array=w4106, index (col)=w4108) -> (element=w4090:dbl[])  [unwired: 1 in]
              "Stbd 120" <- w4090
              n301 = Index Array(array=w4105, index (col)=w4111) -> (element=w4092:dbl[])  [unwired: 1 in]
              "Corners 60" <- w4092
              n302 = Index Array(array=w4107, index (col)=w4108) -> (element=w4091:dbl[])  [unwired: 1 in]
              "Port 120" <- w4091
              n303 = Index Array(array=w4106, index (col)=w4111) -> (element=w4093:dbl[])  [unwired: 1 in]
              "Stbd 60" <- w4093
              n304 = Index Array(array=w4107, index (col)=w4111) -> (element=w4094:dbl[])  [unwired: 1 in]
              "Port 60" <- w4094
              n305 = case shown="\"Simulated Signals Ohio\"" w4086 {
                tunnel: [w4121 w4129 w4137] -> w4104
                tunnel: [w4120 w4128 w4136] -> w4099
                tunnel: w4094 -> [w4119 w4127 w4135]
                tunnel: w4093 -> [w4118 w4126 w4134]
                tunnel: w4092 -> [w4117 w4125 w4133]
                frame "Ohio Class" {
                  w4120 = sgl[] [1.0, 2.0, 3.0, 4.0, 5.0, 6.0, 7.0, 8.0, 9.0, 10.0, 11.0, 12.0, 13.0, 14.0, 15.0, 16.0, 17.0, 18.0, 19.0, 20.0, 21.0, 22.0, 23.0, 24.0, 25.0, 26.0, 27.0, 28.0, 29.0, 30.0]  # Sensor Number
                  n306 = Insert Into Array "Start with Corners,\nadd Stbd Accels"(array=w4117, index=12, new element=w4118) -> (w4123:dbl[])
                  n307 = Insert Into Array "Add Port Accels"(array=w4123, index=21, new element=w4119) -> (w4121:dbl[])
                }
                frame "LA Class" {
                  w4128 = sgl[] [1.0, 2.0, 3.0, 4.0, 5.0, 6.0, 7.0, 8.0, 9.0, 10.0, 11.0, 12.0, 13.0, 14.0, 15.0, 16.0, 17.0, 18.0, 19.0, 20.0, 21.0, 22.0, 23.0, 24.0, 25.0, 26.0, 27.0, 28.0, 29.0, 30.0, 31.0, 32.0, 33.0, 34.0, 35.0, 36.0]  # Sensor Number
                  n308 = Insert Into Array "Start with Corners,\nadd Stbd Accels"(array=w4125, index=12, new element=w4126) -> (w4131:dbl[])
                  n309 = Insert Into Array "Add Port Accels"(array=w4131, index=24, new element=w4127) -> (w4129:dbl[])
                }
                frame "Simulated Signals Ohio" {
                  w4136 = sgl[] [1.0, 2.0, 3.0, 4.0, 5.0, 6.0, 7.0, 8.0, 9.0, 10.0, 11.0, 12.0, 13.0, 14.0, 15.0, 16.0, 17.0, 18.0, 19.0, 20.0, 21.0, 22.0, 23.0, 24.0, 25.0, 26.0, 27.0, 28.0, 29.0, 30.0]  # Sensor Number
                  n310 = Insert Into Array "Start with Corners,\nadd Stbd Accels"(array=w4133, index=12, new element=w4134) -> (w4139:dbl[])
                  n311 = Insert Into Array "Add Port Accels"(array=w4139, index=21, new element=w4135) -> (w4137:dbl[])
                }
              }
              n312 = Index Array(array=w4105, index (col)=w4108) -> (element=w4089:dbl[])  [unwired: 1 in]
              "Corners 120" <- w4089
              n313 = case shown="True" "Save BG" {
                tunnel: w4094 -> [_ w4174]
                tunnel: w4093 -> [_ w4175]
                tunnel: w4092 -> [_ w4173]
                tunnel: w4091 -> [_ w4168]
                tunnel: w4090 -> [_ w4169]
                tunnel: w4089 -> [_ w4170]
                frame False {
                }
                frame True {
                  w4155 = string[][] []
                  n314 = local read "Boat File"() -> (w4146:path)
                  n315 = Array Size(array=w4173) -> (size(s)=w4172:i32)
                  n316 = Array Size(array=w4170) -> (size(s)=w4171:i32)
                  n317 = call <vilib>:"New Report.vi"("report type"=T11."Excel", "template (empty)"=w4146) -> ("report out"=w4167:refnum<class "NI_report.lvclass">, "error out"=w4166:errorcluster)  [unwired: 12 in]
                  n318 = Insert Into Array(array=w4173, index=w4172, new element #1=w4175, new element #2=w4174) -> (w4161:dbl[])
                  n319 = Insert Into Array(array=w4170, index=w4171, new element #1=w4169, new element #2=w4168) -> (w4157:dbl[])
                  n320 = call <vilib>:"Excel Get Worksheet.vi"("report in"=w4167, "worksheet index (0)"=3, "error in (no error)"=w4166) -> ("report out"=w4164:refnum<class "NI_report.lvclass">, "error out"=w4163:errorcluster)  [unwired: 11 out]
                  n321 = Number To Fractional String(number=w4161, precision (6)=i16 3 ("width (-)")) -> (F-format string=w4160:string[])  [unwired: 2 in]
                  n322 = Number To Fractional String(number=w4157, precision (6)=i16 3 ("width (-)")) -> (F-format string=w4156:string[])  [unwired: 2 in]
                  n323 = Insert Into Array(array=w4155, new element=w4160) -> (w4150:string[][])  [unwired: 2 in]
                  n324 = Insert Into Array(array=w4155, new element=w4156) -> (w4148:string[][])  [unwired: 2 in]
                  n325 = Transpose 2D Array(2D array=w4150) -> (transposed array=w4149:string[][])
                  n326 = call-poly <vilib>:"Excel Easy Table.vi"("report in"=w4164, "start (0, 0)"=cluster{"row":i32, "column":i32} {"row"=1, "column"=3}, "text data"=w4149, "error in (no error)"=w4163) -> ("report out"=w4152:refnum<class "NI_report.lvclass">, "error out"=w4153:errorcluster)  [unwired: 7 in, 3 out]
                  n327 = Transpose 2D Array(2D array=w4148) -> (transposed array=w4147:string[][])
                  n328 = call-poly <vilib>:"Excel Easy Table.vi"("report in"=w4152, "start (0, 0)"=cluster{"row":i32, "column":i32} {"row"=1, "column"=4}, "text data"=w4147, "error in (no error)"=w4153) -> ("report out"=w4145:refnum<class "NI_report.lvclass">, "error out"=w4144:errorcluster)  [unwired: 7 in, 3 out]
                  n329 = call <vilib>:"Excel Set Cell Font.vi"("report in"=w4145, "font"=T18 {"font name"="Calibri", "font size"=12.0, "bold"=0, "italic"=0, "underline"=0, "strike through"=0, "font color"=16777216}, "error in (no error)"=w4144) -> ("report out"=w4142:refnum<class "NI_report.lvclass">, "error out"=w4141:errorcluster)  [unwired: 11 in]
                  n330 = call-dynamic "Save Report to File.vi"("report in"=w4142, "report file path"=w4146, "error in (no error)"=w4141) -> ()  [unwired: 11 in, 2 out]
                }
              }
              n331 = Bundle("Sensor Number"=w4099, w4104) -> (w4103:cluster{"Sensor Number":sgl[], dbl[]})  [unwired: 1 in]
              n332 = Initialize Array(w4103, 1 ("dimension size")) -> (→"XY Graph":cluster{"Sensor Number":sgl[], dbl[]}[])
            }
          }
          n333 = Not(x=w3568) -> (.not. x?=w3567:bool)
          n334 = local read "Ship Class"() -> (w3475:T4)
          n335 = case shown="False" "Automarker" {
            tunnel: [FALSE w3865] -> w3366
            frame False {
            }
            frame True {
              n336 = call "Elapsed Time"("Time Target (s)"="Marker Seconds") -> ("Time has Elapsed"=w3866:bool)  [unwired: 11 in, 7 out]
              n337 = case shown="False" w3866 {
                tunnel: [FALSE TRUE] -> w3865
                frame False {
                }
                frame True {
                }
              }
            }
          }
          n338 = case shown="\"LA Class\"" w3475 {
            tunnel: w3333 -> [w4182 w4200 w4216]
            tunnel: w3332 -> [w4177 w4198 w4214]
            tunnel: w3331 -> [w4190 w4203 w4219]
            tunnel: w3330 -> [w4191 w4207 w4223]
            tunnel: [w4176 w4192 w4208] -> w3334
            frame "Simulated Signals Ohio", Default {
              n339 = Array Size(array=w4190) -> (size(s)=w4188:i32[])
              n340 = Index Array(array=w4188, index=1) -> (element=w4187:i32)
              n341 = Insert Into Array(array=w4190, index (dim 1)=w4187, new element=w4191) -> (w4184:dbl[][][])  [unwired: 2 in]
              n342 = Array Size(array=w4184) -> (size(s)=w4186:i32[])
              n343 = Index Array(array=w4186, index=1) -> (element=w4183:i32)
              n344 = Insert Into Array(array=w4184, index (dim 1)=w4183, new element=w4182) -> (w4178:dbl[][][])  [unwired: 2 in]
              n345 = Array Size(array=w4178) -> (size(s)=w4180:i32[])
              n346 = Index Array(array=w4180, index=1) -> (element=w4179:i32)
              n347 = Insert Into Array(array=w4178, index (dim 1)=w4179, new element=w4177) -> (w4176:dbl[][][])  [unwired: 2 in]
            }
            frame "LA Class" {
              n348 = Array Size(array=w4200) -> (size(s)=w4201:i32[])
              n349 = Array Size(array=w4203) -> (size(s)=w4206:i32[])
              n350 = Index Array(array=w4201, index=1) -> (element=w4199:i32)
              n351 = Index Array(array=w4206, index=1) -> (element=w4204:i32)
              n352 = Insert Into Array(array=w4200, index (dim 1)=w4199, new element=w4198) -> (w4193:dbl[][][])  [unwired: 2 in]
              n353 = Insert Into Array(array=w4203, index (dim 1)=w4204, new element=w4207) -> (w4194:dbl[][][])  [unwired: 2 in]
              n354 = Array Size(array=w4194) -> (size(s)=w4197:i32[])
              n355 = Index Array(array=w4197, index=1) -> (element=w4195:i32)
              n356 = Insert Into Array(array=w4194, index (dim 1)=w4195, new element=w4193) -> (w4192:dbl[][][])  [unwired: 2 in]
            }
            frame "Ohio Class" {
